vi "hybrid Connect to Control.vi"(1 "error in":errorcluster) -> (2 "VI Refnum":refnum<vi>, 3 "Success":bool, 4 "error out":errorcluster)   [LabVIEW 2019]
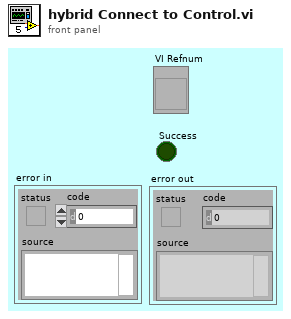
[diagram p1: front panel]
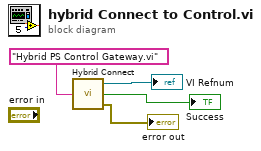
[diagram p0: block diagram]
diagram:
  n1 = call "Hybrid Connect.vi"("VI Name"="Hybrid PS Control Gateway.vi") -> ("VI Refnum"=→"VI Refnum":refnum<vi>, "Success"=→"Success":bool, "error out"=→"error out":errorcluster)
